vi "N-Parametric Double FFT Mesurament RT.vi"(8 "Triangular Multiply Factor":dbl[](array[numeric])=[1.0, 0.8, 0.95, 0.85, 0.9], 9 "Enable triangular scaling":bool=TRUE, 10 "Triangolo dritto?":bool, 11 "#Signals":u32(slide)=5 scale=1.0..5.0) -> ()   [LabVIEW 2014]
uses:
  <vilib>/Platform/TimedLoop/XDataNode/timing_clust.ctl
  <vilib>/Platform/TimedLoop/XDataNode/nitl_modes.ctl
  <vilib>/Platform/TimedLoop/XDataNode/wakeup.ctl
  <vilib>/FPGAPlugInAG/sbRIO-9636/niLvFpga_Open_sbRIO-9636.vi
  <vilib>/rvi/interface/common/dynamic/niFpgaDynamicAddResources.vi
  <vilib>/FPGAPlugInAG/Dynamic/niLvFpga_Reset_Dynamic.vi
  <vilib>/Utility/error.llb/Error Cluster From Error Code.vi
  <vilib>/rvi/errors/niLvFpgaAdjustHostInterfaceError.vi
  <vilib>/rvi/interface/common/niFpgaWaitOnOcc.vi
  <vilib>/FPGAPlugInAG/Dynamic/niLvFpga_Run_Dynamic.vi
  <vilib>/FPGAPlugInAG/Dynamic/niLvFpga_Abort_Dynamic.vi
  <vilib>/FPGAPlugInAG/Dynamic/niLvFpga_Close_Dynamic.vi
  <vilib>/rvi/interface/nirviOpenFPGA/nirviOpenFPGA.xnode
  FPGA Bitfiles/LaserDistanceSen_FPGATarget_N-ParametricDoub_YVLbjAYtdP4.lvbitx
  FPGA Target/Test VIs/N-Parametric Double FFT Mesurament Test.vi
  FPGA Bitfiles/LaserDistanceSen_FPGATarget_N-ParametricDoub_qx5IM88U9d4.lvbitx
  FPGA Target/Test VIs/N-Parametric Double FFT Mesurament Test SLOW.vi
  <vilib>/rvi/interface/nirviMethod/nirviMethod.xnode
  <vilib>/rvi/interface/nirviReadWriteControl/nirviReadWriteControl.xnode
  <vilib>/Platform/TimedLoop/XDataNode/XDataNode.xnode
  <vilib>/rvi/interface/nirviCloseFPGA/nirviCloseFPGA.xnode
  <vilib>/FPGAPlugInAG/Dynamic/niLvFpga_ConfigureFifo_Dynamic.vi
  <vilib>/rvi/errors/niLvFpgaMergeErrorWithErrorCode.vi
  <vilib>/FPGAPlugInAG/Dynamic/niLvFpga_StartFifo_Dynamic.vi
  <vilib>/rvi/interface/Simulation/niFpgaSimulationCallBeginRW.vi
  <vilib>/FPGAPlugInAG/Dynamic/niLvFpga_ReadFifo_Dynamic.vi
  <vilib>/Platform/TimedLoop/XDataNode/XDNodeRunTimeDep.lvlib
  NiFpgaLv.dll
panel:
  in  "Sample /Modulation Frequency":enum32{"40MHz/32KHz", "30MHz/24Khz"}(radio)
  out "current sig factor":u32
  out "mean factor 1":dbl[](array[numeric])=[1.0, 0.7647004729921506, 0.9587386483466616, 0.823312577391412, 0.8946731320619146]
  out "mean factor 2":dbl[](array[numeric])=[0.9613248197180021, 0.8004726992011919, 0.9202842728499455, 0.8411537208279052, 0.8795877616861416]
  in  "#measure for factor":u32=10
  in  "indice della triangolare a fattore 1":i32
  out "Freq correction factor 1":dbl[](array[numeric])
  out "Freq correction factor 2":dbl[](array[numeric])
  out "Frequencies 2":dbl[](array[numeric])
  out "Frequencies 1":dbl[](array[numeric])
  in  "tieni premuto per":i32=1
  out "Second Std Deviations %":dbl[](array[numeric])
  out "First Std Deviations %":dbl[](array[numeric])
  out "Second Mean Freq Curves":dbl[][](graph)
  out "First Mean Freq Curves":dbl[][](graph)
  in  "# Measurements for Linearization":i32=10
  out "Current Signal":i32
  in  "Linearization?":bool
  out "Second Edge N-FFT":dbl[](graph)
  out "First Edge N-FFT":dbl[](graph)
  in  "stop":bool
  in  "Initial Latency points":u32(slide) scale=0.0..1249.0
  out "Elements Remaining FFT":u32
  out "Elements Remaining Signal":u32
  out "N-Signals":dbl[](graph)
  in  "Snapshot":bool
  in  "Windowing":T1(ring)
  in  "first bin":i32=5
  in  "last bin":i32=255
  in  "lower limit 2":u32(slide)=738 scale=625.0..738.0
  in  "lower limit 1":u32(slide)=113 scale=0.0..113.0
  # "OFFLINE parameters"
  # "WARNING:\nOnce pressed wait untill the end of operation"
  # "Max Detection FFT bin range"
  # "ONLINE parameters"
  # "Calcolo del fattore correttivo di frequenza"
  # "1"
  # "1"
  # "0,82"
  # "0,76"
  # "0,95"
  # "0,96"
  # "0,87"
  # "0,82"
  # "0,91"
  # "0,90"
  # "1st triangular"
  # "2nd triangular"
  # "3rd triangular"
  # "4th triangular"
  # "5th triangular"
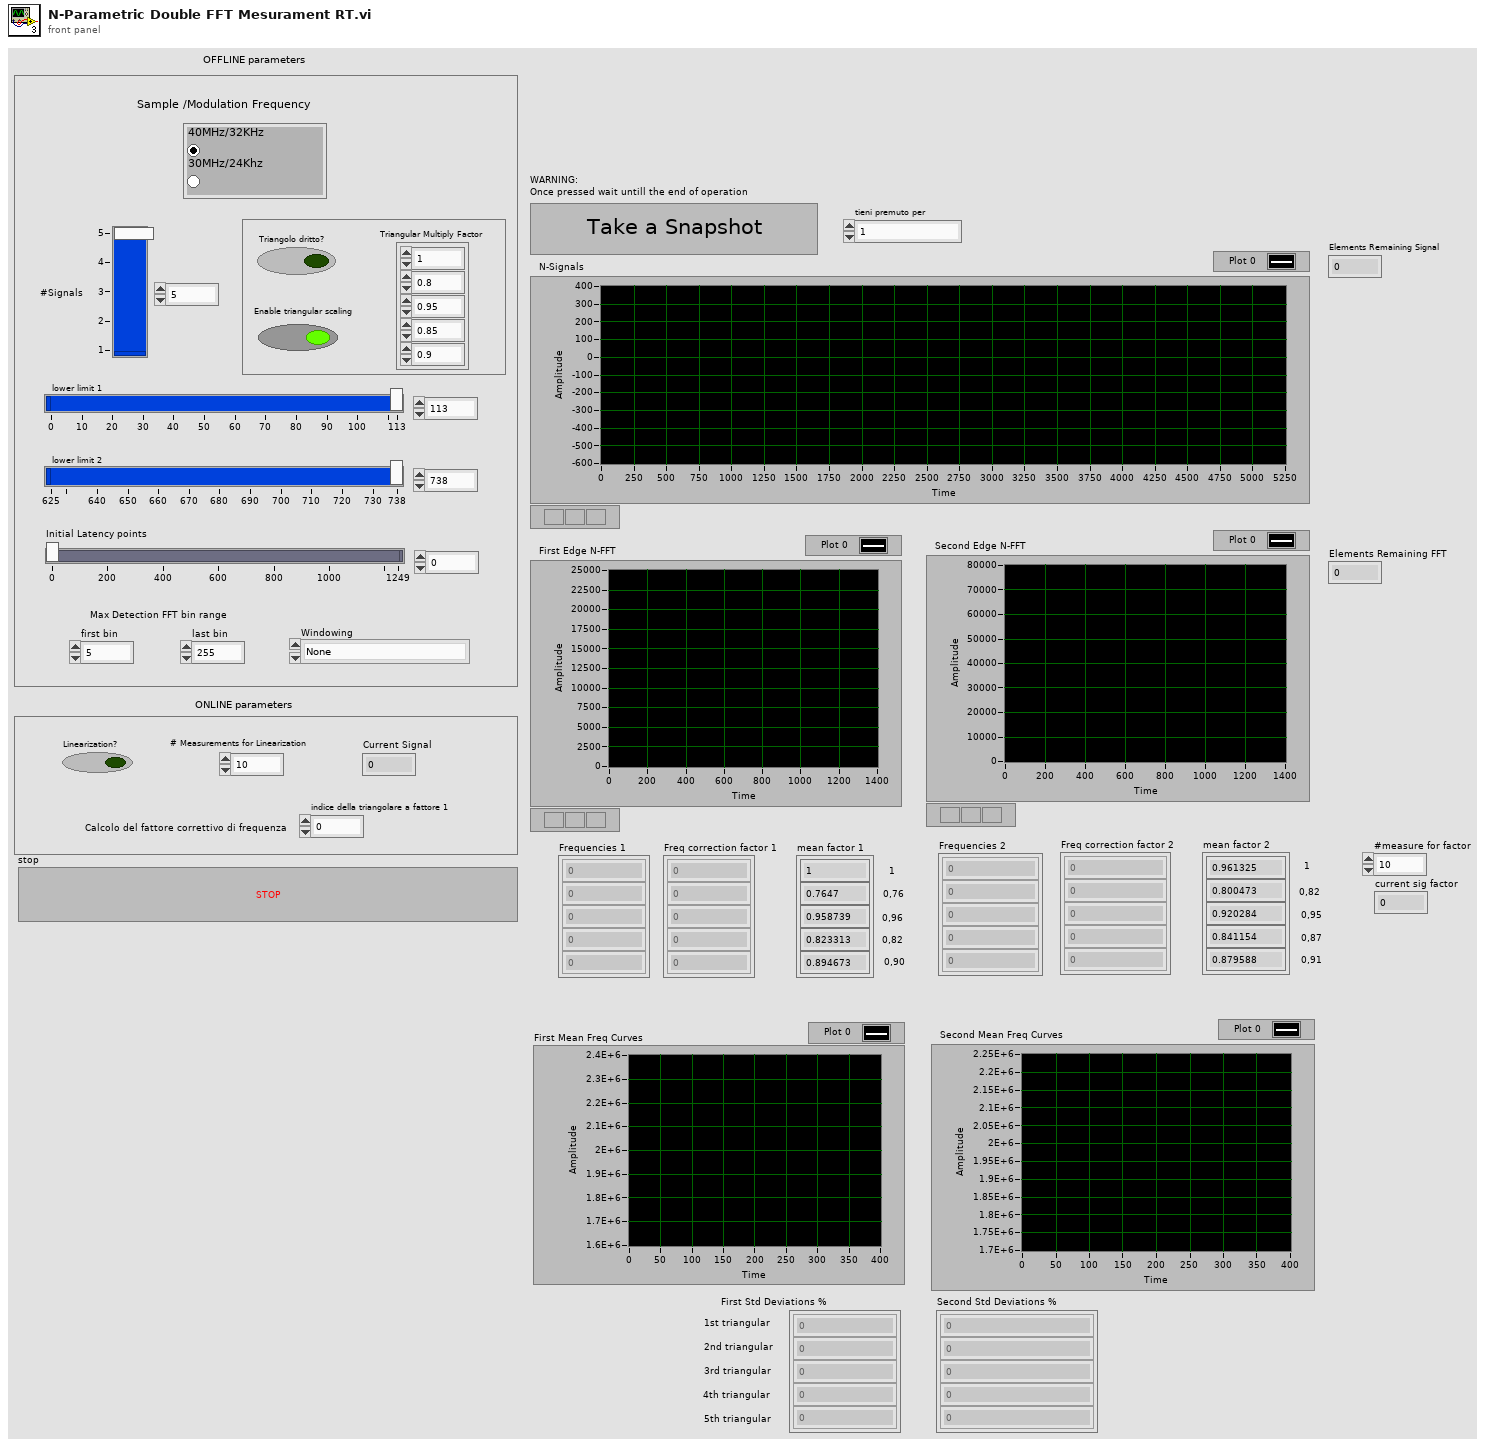
[diagram p1: front panel]
types:
  T1 = enum16{"None", "Hanning", "Hamming", "Blackman", "Blackman-Harris"}
  T2 = typedef "XDNodeRunTimeDep.lvlib/timing_clust.ctl" = cluster{"Expected End [f-1]":u64, "Actual End [f-1]":u64, "Finished Late? [f-1]":bool, "Expected End [i-1]":u64, "Actual End [i-1]":u64, "Finished Late? [i-1]":bool, "Expected Start [i]":u64, "Actual Start [i]":u64, "Expected Start [f]":u64, "Actual Start [f]":u64, "Source Name":string, "Structure Name":string, "Period":i64, "Deadline":i64, "Offset":i64, "Start":i64, "Priority":i32, "Timeout":i32, "Mode":T3, "Wakeup Reason":T4, "Error":errorcluster, "Source Type":string, "Secondary Source Type":string, "Global End Time":u64, "Global Start Time":u64, "Frame Duration":u64, "Iteration Duration":u64, "Assigned CPU":i32, "I/O Scan Engine Mode":u32}
  T3 = typedef "XDNodeRunTimeDep.lvlib/nitl_modes.ctl" = enum32{"No Change", "Process missed periods, maintain original phase", "Discard missed periods, maintain original phase", "Process missed periods, ignore original phase", "Discard missed periods, ignore original phase"}
  T4 = typedef "XDNodeRunTimeDep.lvlib/wakeup.ctl" = enum32{"Normal", "Aborted", "Asynchronous wakeup", "Timing source error", "Timed loop error", "Timeout"}
  T5 = typedef "NI_Matrix.lvlib/RealMatrix.ctl" = dbl[][]
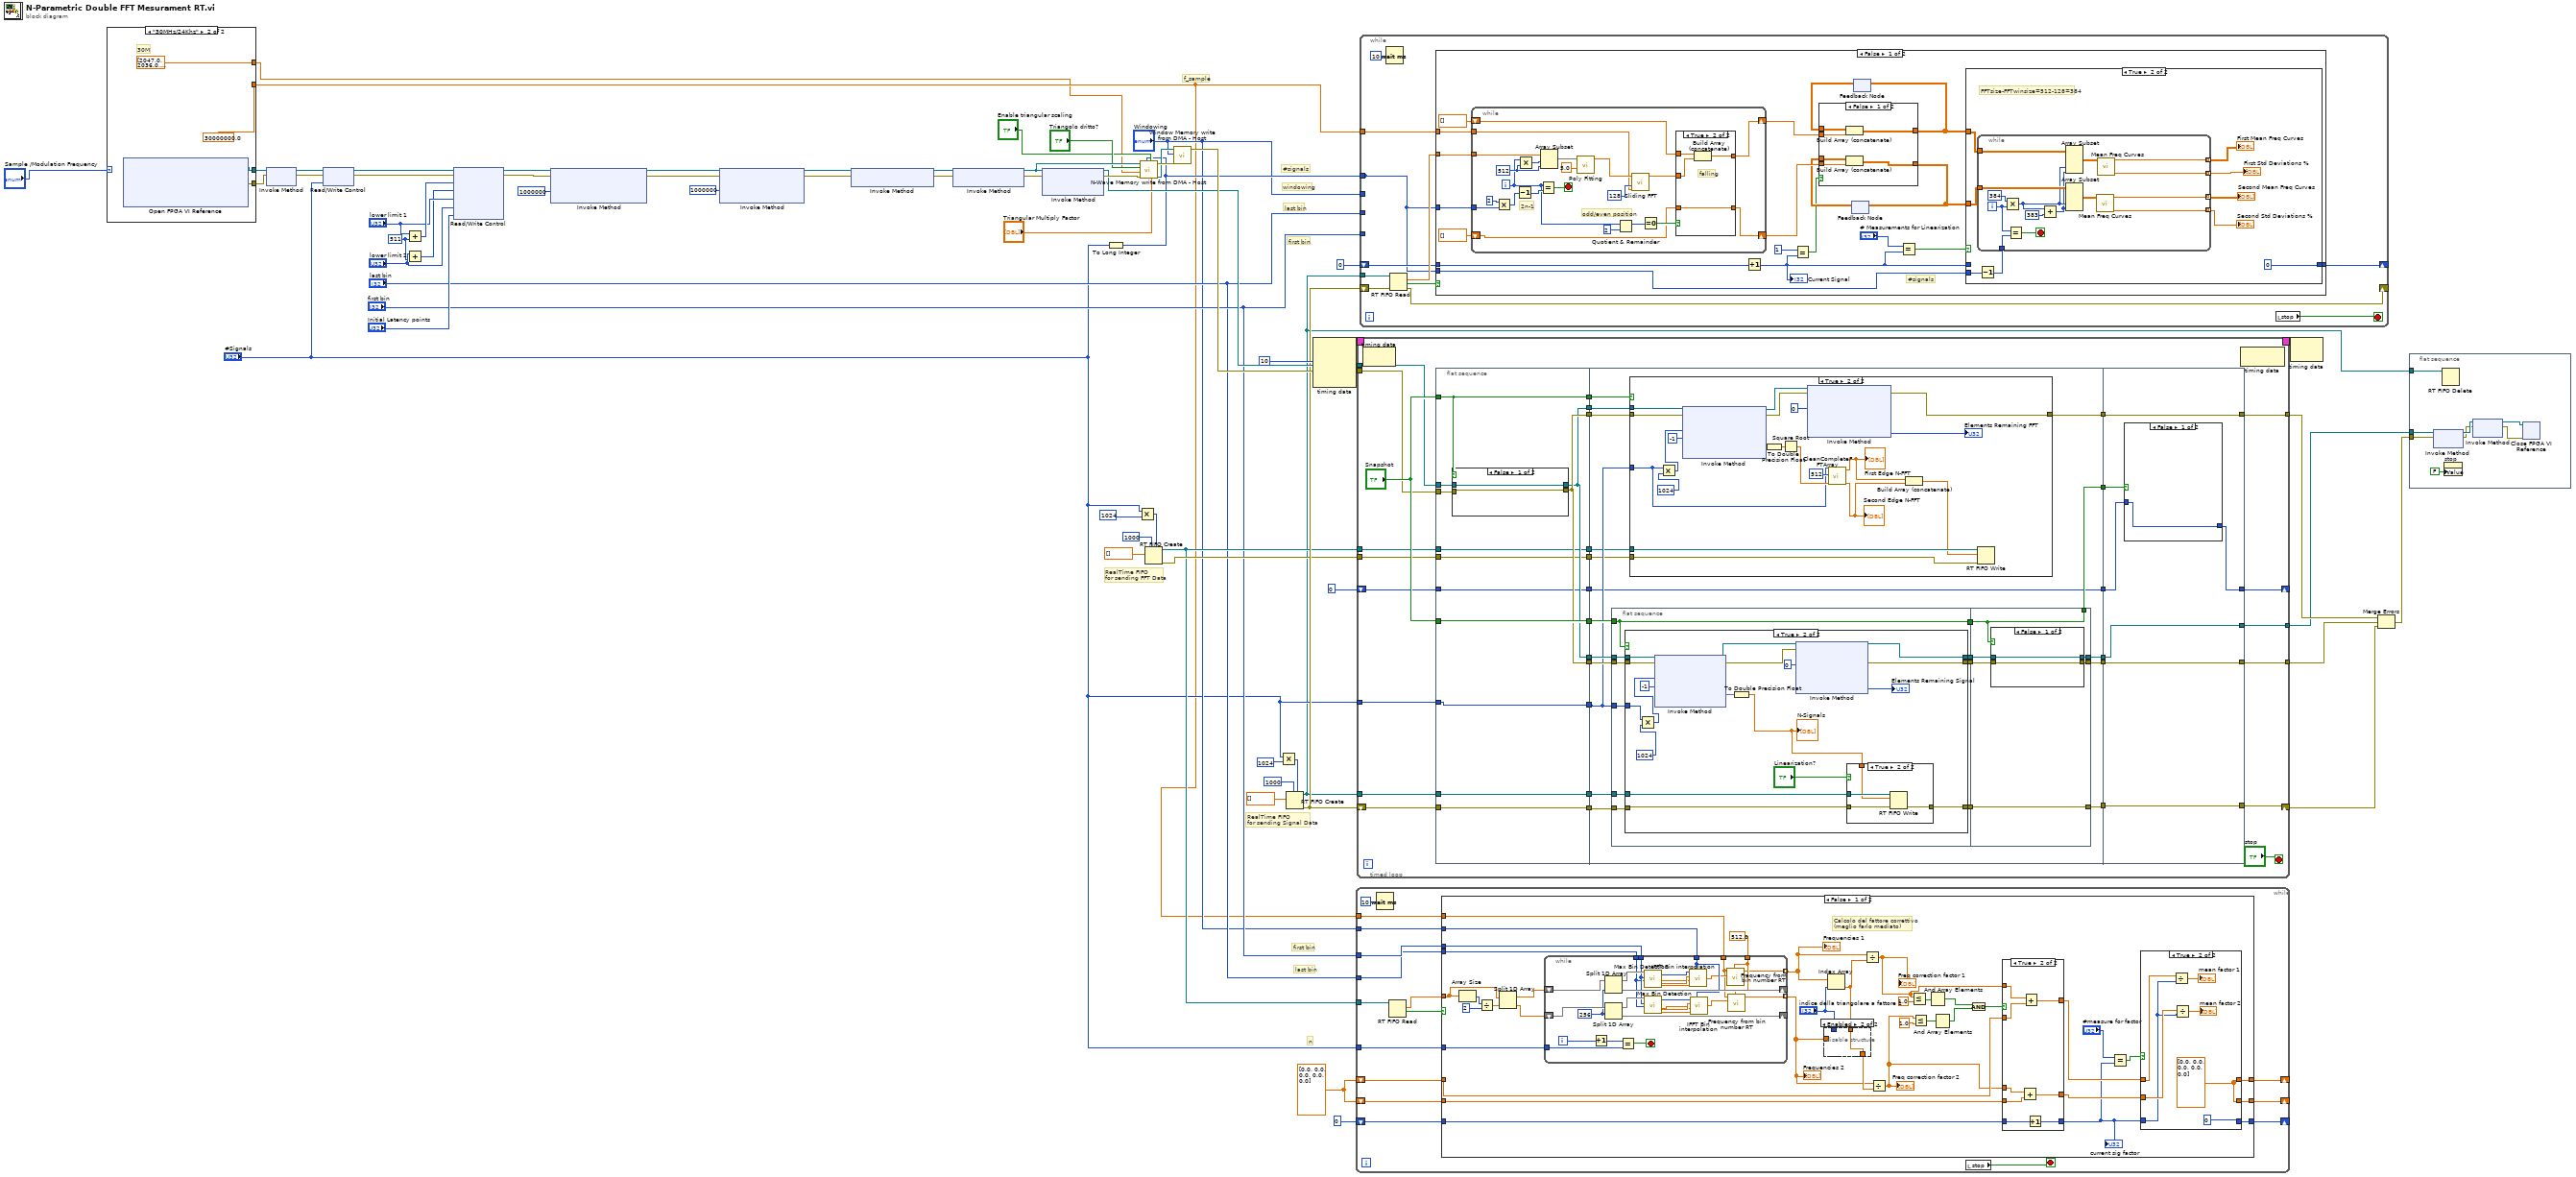
[diagram p0: block diagram]
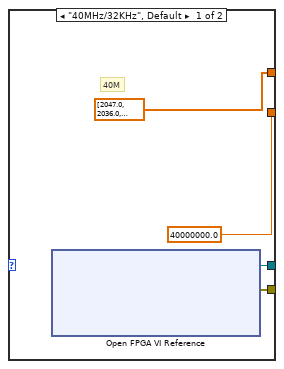
[diagram p2: hidden frame]
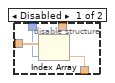
[diagram p3: hidden frame]
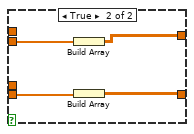
[diagram p8: hidden frame]
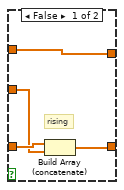
[diagram p9: hidden frame]
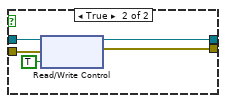
[diagram p11: hidden frame]
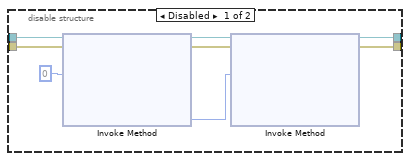
[diagram p13: hidden frame]
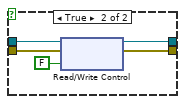
[diagram p15: hidden frame]
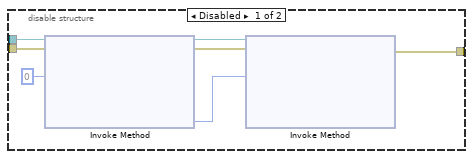
[diagram p17: hidden frame]
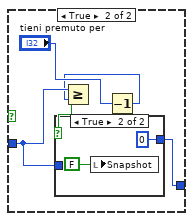
[diagram p18: hidden frame]
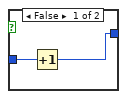
[diagram p19: hidden frame]
diagram:
  w4 = dbl[] [0.0, 0.0, 0.0, 0.0, 0.0] ("second subarray")
  w60 = u32 511 ("y")
  # "n"
  # "last bin"
  # "first bin"
  # "RealTime FIFO \nfor sending FFT Data"
  # "f_sample"
  # "#signals"
  # "RealTime FIFO \nfor sending Signal Data"
  # "windowing"
  # "last bin"
  # "first bin"
  n1 = case shown="\"30MHz/24Khz\"" "Sample /Modulation Frequency" {
    tunnel: [w68 w71] -> w34
    tunnel: [w67 w72] -> w33
    tunnel: [40000000.0 ("Sample Rate (S/s)") 30000000.0 ("Sample Rate (S/s)")] -> w2
    tunnel: [dbl[] [2047.0, 2036.0, 2024.0, 2013.0, 2002.0, 1990.0, 1979.0, 1968.0, 1956.0, 1945.0, 1934.0, 1923.0, 1912.0, 1900.0, 1889.0, 1878.0, 1867.0, 1856.0, 1845.0, 1833.0, 1822.0, 1811.0, 1800.0, 1789.0, 1778.0, 1767.0, 1756.0, 1745.0, 1734.0, 1723.0, 1712.0, 1702.0, 1691.0, 1680.0, 1669.0, 1658.0, 1647.0, 1636.0, 1626.0, 1615.0, 1604.0, 1593.0, 1583.0, 1572.0, 1561.0, 1550.0, 1540.0, 1529.0, 1518.0, 1508.0, 1497.0, 1487.0, 1476.0, 1465.0, 1455.0, 1444.0, 1434.0, 1423.0, 1413.0, 1402.0, 1392.0, 1381.0, 1371.0, 1360.0, 1350.0, 1340.0, 1329.0, 1319.0, 1309.0, 1298.0, 1288.0, 1278.0, 1267.0, 1257.0, 1247.0, 1237.0, 1226.0, 1216.0, 1206.0, 1196.0, 1186.0, 1176.0, 1165.0, 1155.0, 1145.0, 1135.0, 1125.0, 1115.0, 1105.0, 1095.0, 1085.0, 1075.0, 1065.0, 1055.0, 1045.0, 1035.0, 1025.0, 1015.0, 1006.0, 996.0, 986.0, 976.0, 966.0, 956.0, 947.0, 937.0, 927.0, 917.0, 908.0, 898.0, 888.0, 879.0, 869.0, 859.0, 850.0, 837.0, 826.0, 816.0, 804.0, 796.0, 788.0, 778.0, 769.0, 758.0, 750.0, 743.0, 733.0, 724.0, 717.0, 709.0, 701.0, 693.0, 686.0, 677.0, 669.0, 661.0, 653.0, 645.0, 638.0, 630.0, 622.0, 615.0, 607.0, 599.0, 592.0, 583.0, 576.0, 569.0, 561.0, 554.0, 547.0, 539.0, 532.0, 525.0, 518.0, 509.0, 501.0, 492.0, 486.0, 478.0, 471.0, 463.0, 456.0, 450.0, 442.0, 435.0, 429.0, 421.0, 415.0, 408.0, 401.0, 394.0, 388.0, 381.0, 375.0, 368.0, 361.0, 355.0, 349.0, 342.0, 336.0, 330.0, 323.0, 317.0, 311.0, 304.0, 298.0, 292.0, 286.0, 279.0, 273.0, 267.0, 261.0, 255.0, 249.0, 242.0, 236.0, 230.0, 224.0, 218.0, 212.0, 206.0, 200.0, 194.0, 187.0, 181.0, 175.0, 169.0, 163.0, 157.0, 150.0, 144.0, 138.0, 132.0, 125.0, 119.0, 113.0, 107.0, 101.0, 95.0, 88.0, 82.0, 77.0, 71.0, 65.0, 59.0, 53.0, 47.0, 41.0, 35.0, 29.0, 23.0, 18.0, 11.0, 6.0, 0.0, -6.0, -12.0, -18.0, -23.0, -29.0, -35.0, -41.0, -47.0, -52.0, -58.0, -64.0, -69.0, -75.0, -81.0, -87.0, -92.0, -98.0, -104.0, -109.0, -115.0, -121.0, -126.0, -132.0, -138.0, -144.0, -149.0, -155.0, -161.0, -166.0, -172.0, -177.0, -183.0, -189.0, -194.0, -200.0, -205.0, -211.0, -216.0, -222.0, -227.0, -233.0, -238.0, -244.0, -249.0, -255.0, -260.0, -266.0, -271.0, -277.0, -283.0, -288.0, -294.0, -299.0, -304.0, -310.0, -315.0, -321.0, -326.0, -331.0, -337.0, -342.0, -348.0, -353.0, -358.0, -364.0, -369.0, -375.0, -380.0, -385.0, -391.0, -396.0, -402.0, -407.0, -413.0, -418.0, -423.0, -429.0, -434.0, -439.0, -445.0, -450.0, -456.0, -461.0, -466.0, -472.0, -477.0, -483.0, -488.0, -493.0, -499.0, -504.0, -510.0, -515.0, -520.0, -526.0, -531.0, -537.0, -542.0, -548.0, -553.0, -558.0, -564.0, -569.0, -574.0, -580.0, -585.0, -590.0, -596.0, -601.0, -606.0, -612.0, -617.0, -622.0, -628.0, -633.0, -638.0, -644.0, -649.0, -654.0, -660.0, -665.0, -670.0, -676.0, -681.0, -686.0, -692.0, -697.0, -702.0, -708.0, -713.0, -718.0, -723.0, -729.0, -734.0, -739.0, -744.0, -750.0, -755.0, -760.0, -765.0, -771.0, -776.0, -781.0, -786.0, -792.0, -797.0, -802.0, -807.0, -812.0, -818.0, -823.0, -828.0, -833.0, -839.0, -844.0, -849.0, -854.0, -859.0, -865.0, -870.0, -875.0, -880.0, -885.0, -891.0, -896.0, -901.0, -906.0, -911.0, -916.0, -922.0, -927.0, -932.0, -937.0, -943.0, -948.0, -953.0, -958.0, -963.0, -969.0, -974.0, -979.0, -984.0, -989.0, -995.0, -1000.0, -1005.0, -1010.0, -1015.0, -1021.0, -1026.0, -1031.0, -1036.0, -1041.0, -1047.0, -1052.0, -1057.0, -1062.0, -1067.0, -1073.0, -1078.0, -1083.0, -1088.0, -1093.0, -1099.0, -1104.0, -1109.0, -1114.0, -1119.0, -1124.0, -1130.0, -1135.0, -1140.0, -1145.0, -1150.0, -1156.0, -1161.0, -1166.0, -1171.0, -1176.0, -1182.0, -1187.0, -1192.0, -1197.0, -1202.0, -1207.0, -1213.0, -1218.0, -1223.0, -1228.0, -1233.0, -1238.0, -1244.0, -1249.0, -1254.0, -1259.0, -1264.0, -1269.0, -1275.0, -1280.0, -1285.0, -1290.0, -1295.0, -1300.0, -1305.0, -1311.0, -1316.0, -1321.0, -1326.0, -1331.0, -1336.0, -1342.0, -1347.0, -1352.0, -1357.0, -1362.0, -1367.0, -1372.0, -1378.0, -1383.0, -1388.0, -1393.0, -1398.0, -1403.0, -1408.0, -1414.0, -1419.0, -1424.0, -1429.0, -1434.0, -1439.0, -1444.0, -1450.0, -1455.0, -1460.0, -1465.0, -1470.0, -1475.0, -1480.0, -1486.0, -1491.0, -1496.0, -1501.0, -1506.0, -1511.0, -1516.0, -1522.0, -1527.0, -1532.0, -1537.0, -1542.0, -1547.0, -1552.0, -1558.0, -1563.0, -1568.0, -1573.0, -1578.0, -1583.0, -1588.0, -1593.0, -1599.0, -1604.0, -1609.0, -1614.0, -1619.0, -1624.0, -1629.0, -1634.0, -1640.0, -1645.0, -1650.0, -1655.0, -1660.0, -1665.0, -1670.0, -1675.0, -1681.0, -1686.0, -1691.0, -1696.0, -1701.0, -1706.0, -1711.0, -1716.0, -1722.0, -1727.0, -1732.0, -1737.0, -1742.0, -1747.0, -1752.0, -1757.0, -1762.0, -1768.0, -1773.0, -1778.0, -1783.0, -1788.0, -1793.0, -1798.0, -1803.0, -1808.0, -1814.0, -1819.0, -1824.0, -1829.0, -1834.0, -1839.0, -1844.0, -1849.0, -1854.0, -1859.0, -1865.0, -1870.0, -1875.0, -1880.0, -1885.0, -1890.0, -1895.0, -1900.0, -1905.0, -1911.0, -1916.0, -1921.0, -1926.0, -1931.0, -1936.0, -1941.0, -1946.0, -1951.0, -1956.0, -1961.0, -1967.0, -1972.0, -1977.0, -1982.0, -1987.0, -1992.0, -1997.0, -2002.0, -2007.0, -2012.0, -2017.0, -2023.0, -2028.0, -2033.0, -2038.0, -2043.0, -2048.0, -2047.0, -2034.0, -2021.0, -2009.0, -1996.0, -1983.0, -1970.0, -1957.0, -1945.0, -1932.0, -1919.0, -1907.0, -1894.0, -1881.0, -1869.0, -1856.0, -1844.0, -1831.0, -1819.0, -1806.0, -1794.0, -1781.0, -1769.0, -1757.0, -1744.0, -1732.0, -1719.0, -1707.0, -1695.0, -1682.0, -1670.0, -1658.0, -1646.0, -1634.0, -1621.0, -1609.0, -1597.0, -1585.0, -1573.0, -1561.0, -1549.0, -1537.0, -1525.0, -1513.0, -1501.0, -1489.0, -1477.0, -1465.0, -1453.0, -1441.0, -1429.0, -1417.0, -1405.0, -1394.0, -1382.0, -1370.0, -1358.0, -1347.0, -1335.0, -1323.0, -1312.0, -1300.0, -1288.0, -1277.0, -1265.0, -1254.0, -1242.0, -1231.0, -1219.0, -1208.0, -1196.0, -1185.0, -1173.0, -1162.0, -1150.0, -1139.0, -1128.0, -1116.0, -1105.0, -1094.0, -1083.0, -1071.0, -1060.0, -1049.0, -1038.0, -1027.0, -1015.0, -1004.0, -993.0, -982.0, -971.0, -960.0, -949.0, -938.0, -927.0, -916.0, -905.0, -894.0, -883.0, -873.0, -862.0, -851.0, -840.0, -829.0, -819.0, -808.0, -797.0, -786.0, -776.0, -765.0, -754.0, -744.0, -733.0, -722.0, -712.0, -697.0, -685.0, -674.0, -661.0, -652.0, -643.0, -632.0, -622.0, -610.0, -602.0, -594.0, -583.0, -574.0, -566.0, -558.0, -550.0, -542.0, -534.0, -525.0, -516.0, -507.0, -499.0, -491.0, -483.0, -475.0, -467.0, -459.0, -451.0, -443.0, -435.0, -426.0, -419.0, -411.0, -404.0, -396.0, -388.0, -381.0, -373.0, -366.0, -359.0, -349.0, -341.0, -331.0, -325.0, -317.0, -309.0, -301.0, -295.0, -288.0, -280.0, -273.0, -266.0, -259.0, -252.0, -246.0, -239.0, -231.0, -225.0, -219.0, -212.0, -205.0, -199.0, -192.0, -186.0, -180.0, -173.0, -167.0, -161.0, -155.0, -148.0, -142.0, -136.0, -130.0, -124.0, -118.0, -112.0, -106.0, -100.0, -94.0, -88.0, -82.0, -76.0, -70.0, -64.0, -58.0, -52.0, -46.0, -40.0, -34.0, -28.0, -21.0, -15.0, -9.0, -3.0, 2.0, 9.0, 15.0, 21.0, 27.0, 33.0, 39.0, 45.0, 51.0, 57.0, 63.0, 69.0, 75.0, 81.0, 86.0, 92.0, 98.0, 103.0, 110.0, 116.0, 121.0, 127.0, 133.0, 138.0, 144.0, 149.0, 155.0, 161.0, 166.0, 172.0, 177.0, 183.0, 189.0, 194.0, 200.0, 205.0, 211.0, 216.0, 221.0, 227.0, 232.0, 238.0, 243.0, 249.0, 254.0, 259.0, 265.0, 270.0, 276.0, 281.0, 286.0, 292.0, 297.0, 303.0, 308.0, 314.0, 319.0, 324.0, 329.0, 335.0, 340.0, 345.0, 351.0, 356.0, 361.0, 366.0, 371.0, 377.0, 382.0, 387.0, 392.0, 397.0, 403.0, 408.0, 413.0, 418.0, 423.0, 429.0, 434.0, 439.0, 444.0, 449.0, 454.0, 459.0, 464.0, 469.0, 474.0, 479.0, 484.0, 489.0, 494.0, 499.0, 504.0, 509.0, 514.0, 520.0, 525.0, 530.0, 535.0, 540.0, 545.0, 550.0, 555.0, 560.0, 565.0, 570.0, 575.0, 580.0, 585.0, 590.0, 595.0, 600.0, 605.0, 610.0, 615.0, 620.0, 625.0, 630.0, 636.0, 641.0, 646.0, 651.0, 656.0, 661.0, 666.0, 671.0, 676.0, 681.0, 686.0, 691.0, 696.0, 701.0, 706.0, 711.0, 716.0, 721.0, 726.0, 731.0, 736.0, 741.0, 746.0, 751.0, 756.0, 761.0, 765.0, 770.0, 775.0, 780.0, 785.0, 790.0, 795.0, 800.0, 805.0, 810.0, 815.0, 820.0, 825.0, 829.0, 834.0, 839.0, 844.0, 849.0, 854.0, 859.0, 864.0, 868.0, 873.0, 878.0, 883.0, 888.0, 893.0, 897.0, 902.0, 907.0, 912.0, 917.0, 921.0, 926.0, 931.0, 936.0, 941.0, 945.0, 950.0, 955.0, 960.0, 965.0, 969.0, 974.0, 979.0, 984.0, 988.0, 993.0, 998.0, 1003.0, 1007.0, 1012.0, 1017.0, 1022.0, 1027.0, 1031.0, 1036.0, 1041.0, 1046.0, 1051.0, 1055.0, 1060.0, 1065.0, 1070.0, 1075.0, 1079.0, 1084.0, 1089.0, 1094.0, 1098.0, 1103.0, 1108.0, 1113.0, 1118.0, 1122.0, 1127.0, 1132.0, 1137.0, 1141.0, 1146.0, 1151.0, 1156.0, 1161.0, 1165.0, 1170.0, 1175.0, 1180.0, 1184.0, 1189.0, 1194.0, 1199.0, 1204.0, 1208.0, 1213.0, 1218.0, 1223.0, 1227.0, 1232.0, 1237.0, 1242.0, 1246.0, 1251.0, 1256.0, 1261.0, 1265.0, 1270.0, 1275.0, 1280.0, 1284.0, 1289.0, 1294.0, 1299.0, 1303.0, 1308.0, 1313.0, 1318.0, 1322.0, 1327.0, 1332.0, 1336.0, 1341.0, 1346.0, 1351.0, 1355.0, 1360.0, 1365.0, 1370.0, 1374.0, 1379.0, 1384.0, 1388.0, 1393.0, 1398.0, 1403.0, 1407.0, 1412.0, 1417.0, 1421.0, 1426.0, 1431.0, 1436.0, 1440.0, 1445.0, 1450.0, 1454.0, 1459.0, 1464.0, 1469.0, 1473.0, 1478.0, 1483.0, 1487.0, 1492.0, 1497.0, 1502.0, 1506.0, 1511.0, 1516.0, 1520.0, 1525.0, 1530.0, 1535.0, 1539.0, 1544.0, 1549.0, 1553.0, 1558.0, 1563.0, 1567.0, 1572.0, 1577.0, 1582.0, 1586.0, 1591.0, 1596.0, 1600.0, 1605.0, 1610.0, 1614.0, 1619.0, 1624.0, 1628.0, 1633.0, 1638.0, 1643.0, 1647.0, 1652.0, 1657.0, 1661.0, 1666.0, 1671.0, 1675.0, 1680.0, 1685.0, 1689.0, 1694.0, 1699.0, 1703.0, 1708.0, 1713.0, 1717.0, 1722.0, 1727.0, 1731.0, 1736.0, 1741.0, 1746.0, 1750.0, 1755.0, 1760.0, 1764.0, 1769.0, 1774.0, 1778.0, 1783.0, 1788.0, 1792.0, 1797.0, 1802.0, 1806.0, 1811.0, 1816.0, 1820.0, 1825.0, 1830.0, 1834.0, 1839.0, 1844.0, 1848.0, 1853.0, 1858.0, 1862.0, 1867.0, 1871.0, 1876.0, 1881.0, 1885.0, 1890.0, 1895.0, 1899.0, 1904.0, 1909.0, 1913.0, 1918.0, 1923.0, 1927.0, 1932.0, 1937.0, 1941.0, 1946.0, 1951.0, 1955.0, 1960.0, 1965.0, 1969.0, 1974.0, 1978.0, 1983.0, 1988.0, 1992.0, 1997.0, 2002.0, 2006.0, 2011.0, 2016.0, 2020.0, 2025.0, 2029.0, 2034.0, 2039.0, 2043.0, 2048.0] ("Complete SkewTri") dbl[] [2047.0, 2036.0, 2026.0, 2015.0, 2004.0, 1993.0, 1983.0, 1972.0, 1961.0, 1951.0, 1940.0, 1930.0, 1919.0, 1908.0, 1898.0, 1887.0, 1877.0, 1866.0, 1856.0, 1845.0, 1835.0, 1824.0, 1814.0, 1803.0, 1793.0, 1783.0, 1772.0, 1762.0, 1751.0, 1741.0, 1731.0, 1720.0, 1710.0, 1700.0, 1690.0, 1679.0, 1669.0, 1659.0, 1648.0, 1638.0, 1628.0, 1618.0, 1608.0, 1597.0, 1587.0, 1577.0, 1567.0, 1557.0, 1547.0, 1537.0, 1527.0, 1517.0, 1507.0, 1496.0, 1486.0, 1476.0, 1466.0, 1456.0, 1446.0, 1437.0, 1427.0, 1417.0, 1407.0, 1397.0, 1387.0, 1377.0, 1367.0, 1357.0, 1348.0, 1338.0, 1328.0, 1318.0, 1308.0, 1299.0, 1289.0, 1279.0, 1269.0, 1260.0, 1250.0, 1240.0, 1230.0, 1221.0, 1211.0, 1202.0, 1192.0, 1182.0, 1173.0, 1163.0, 1154.0, 1144.0, 1134.0, 1125.0, 1115.0, 1106.0, 1096.0, 1087.0, 1077.0, 1068.0, 1059.0, 1049.0, 1040.0, 1030.0, 1021.0, 1012.0, 1002.0, 993.0, 984.0, 974.0, 965.0, 956.0, 946.0, 937.0, 928.0, 919.0, 909.0, 900.0, 891.0, 882.0, 873.0, 862.0, 853.0, 845.0, 836.0, 827.0, 816.0, 806.0, 797.0, 786.0, 778.0, 769.0, 759.0, 750.0, 742.0, 734.0, 725.0, 717.0, 708.0, 699.0, 691.0, 683.0, 675.0, 668.0, 660.0, 652.0, 645.0, 637.0, 629.0, 622.0, 614.0, 607.0, 599.0, 592.0, 584.0, 577.0, 570.0, 562.0, 555.0, 548.0, 541.0, 534.0, 526.0, 519.0, 512.0, 505.0, 498.0, 491.0, 484.0, 477.0, 470.0, 463.0, 457.0, 449.0, 443.0, 436.0, 429.0, 422.0, 415.0, 409.0, 402.0, 395.0, 388.0, 381.0, 374.0, 367.0, 361.0, 354.0, 347.0, 340.0, 334.0, 327.0, 321.0, 314.0, 308.0, 301.0, 295.0, 288.0, 282.0, 276.0, 269.0, 263.0, 257.0, 251.0, 244.0, 238.0, 232.0, 226.0, 220.0, 213.0, 207.0, 201.0, 195.0, 189.0, 183.0, 177.0, 171.0, 164.0, 158.0, 152.0, 146.0, 140.0, 134.0, 128.0, 122.0, 116.0, 110.0, 104.0, 98.0, 92.0, 86.0, 80.0, 74.0, 68.0, 62.0, 56.0, 50.0, 44.0, 38.0, 32.0, 26.0, 20.0, 15.0, 9.0, 3.0, -3.0, -9.0, -15.0, -21.0, -27.0, -32.0, -38.0, -44.0, -50.0, -56.0, -61.0, -67.0, -73.0, -79.0, -85.0, -90.0, -96.0, -102.0, -108.0, -114.0, -119.0, -125.0, -131.0, -137.0, -142.0, -148.0, -154.0, -159.0, -165.0, -171.0, -176.0, -182.0, -188.0, -193.0, -199.0, -205.0, -210.0, -216.0, -222.0, -227.0, -233.0, -239.0, -244.0, -250.0, -256.0, -261.0, -267.0, -272.0, -278.0, -284.0, -289.0, -295.0, -300.0, -306.0, -311.0, -317.0, -323.0, -328.0, -334.0, -340.0, -345.0, -351.0, -356.0, -362.0, -368.0, -373.0, -379.0, -384.0, -390.0, -395.0, -401.0, -407.0, -412.0, -418.0, -423.0, -429.0, -434.0, -440.0, -445.0, -451.0, -456.0, -462.0, -467.0, -473.0, -478.0, -484.0, -489.0, -495.0, -501.0, -506.0, -512.0, -517.0, -523.0, -528.0, -533.0, -539.0, -544.0, -550.0, -555.0, -561.0, -566.0, -572.0, -577.0, -583.0, -588.0, -594.0, -599.0, -604.0, -610.0, -615.0, -621.0, -626.0, -632.0, -637.0, -642.0, -648.0, -653.0, -659.0, -664.0, -669.0, -675.0, -680.0, -686.0, -691.0, -696.0, -702.0, -707.0, -712.0, -718.0, -723.0, -729.0, -734.0, -739.0, -745.0, -750.0, -755.0, -761.0, -766.0, -771.0, -777.0, -782.0, -787.0, -793.0, -798.0, -803.0, -809.0, -814.0, -819.0, -825.0, -830.0, -835.0, -841.0, -846.0, -851.0, -857.0, -862.0, -868.0, -873.0, -878.0, -884.0, -889.0, -894.0, -900.0, -905.0, -910.0, -916.0, -921.0, -926.0, -932.0, -937.0, -942.0, -947.0, -953.0, -958.0, -963.0, -969.0, -974.0, -979.0, -985.0, -990.0, -995.0, -1001.0, -1006.0, -1011.0, -1017.0, -1022.0, -1027.0, -1033.0, -1038.0, -1043.0, -1048.0, -1054.0, -1059.0, -1064.0, -1070.0, -1075.0, -1080.0, -1086.0, -1091.0, -1096.0, -1102.0, -1107.0, -1112.0, -1118.0, -1123.0, -1128.0, -1134.0, -1139.0, -1144.0, -1149.0, -1155.0, -1160.0, -1165.0, -1171.0, -1176.0, -1181.0, -1186.0, -1192.0, -1197.0, -1202.0, -1208.0, -1213.0, -1218.0, -1223.0, -1229.0, -1234.0, -1239.0, -1245.0, -1250.0, -1255.0, -1260.0, -1266.0, -1271.0, -1276.0, -1281.0, -1287.0, -1292.0, -1297.0, -1302.0, -1308.0, -1313.0, -1318.0, -1323.0, -1329.0, -1334.0, -1339.0, -1344.0, -1350.0, -1355.0, -1360.0, -1365.0, -1371.0, -1376.0, -1381.0, -1386.0, -1392.0, -1397.0, -1402.0, -1407.0, -1412.0, -1418.0, -1423.0, -1428.0, -1433.0, -1439.0, -1444.0, -1449.0, -1454.0, -1460.0, -1465.0, -1470.0, -1475.0, -1480.0, -1486.0, -1491.0, -1496.0, -1501.0, -1507.0, -1512.0, -1517.0, -1522.0, -1528.0, -1533.0, -1538.0, -1543.0, -1548.0, -1554.0, -1559.0, -1564.0, -1569.0, -1575.0, -1580.0, -1585.0, -1590.0, -1595.0, -1601.0, -1606.0, -1611.0, -1616.0, -1622.0, -1627.0, -1632.0, -1637.0, -1642.0, -1648.0, -1653.0, -1658.0, -1663.0, -1668.0, -1674.0, -1679.0, -1684.0, -1689.0, -1695.0, -1700.0, -1705.0, -1710.0, -1715.0, -1721.0, -1726.0, -1731.0, -1736.0, -1741.0, -1747.0, -1752.0, -1757.0, -1762.0, -1767.0, -1773.0, -1778.0, -1783.0, -1788.0, -1793.0, -1799.0, -1804.0, -1809.0, -1814.0, -1819.0, -1825.0, -1830.0, -1835.0, -1840.0, -1845.0, -1851.0, -1856.0, -1861.0, -1866.0, -1871.0, -1877.0, -1882.0, -1887.0, -1892.0, -1897.0, -1903.0, -1908.0, -1913.0, -1918.0, -1923.0, -1929.0, -1934.0, -1939.0, -1944.0, -1949.0, -1955.0, -1960.0, -1965.0, -1970.0, -1975.0, -1981.0, -1986.0, -1991.0, -1996.0, -2001.0, -2007.0, -2012.0, -2017.0, -2022.0, -2027.0, -2032.0, -2038.0, -2043.0, -2048.0, -2047.0, -2035.0, -2022.0, -2010.0, -1997.0, -1985.0, -1973.0, -1960.0, -1948.0, -1936.0, -1923.0, -1911.0, -1899.0, -1887.0, -1874.0, -1862.0, -1850.0, -1838.0, -1826.0, -1814.0, -1801.0, -1789.0, -1777.0, -1765.0, -1753.0, -1741.0, -1729.0, -1717.0, -1705.0, -1693.0, -1681.0, -1670.0, -1658.0, -1646.0, -1634.0, -1622.0, -1610.0, -1599.0, -1587.0, -1575.0, -1563.0, -1552.0, -1540.0, -1528.0, -1517.0, -1505.0, -1494.0, -1482.0, -1470.0, -1459.0, -1447.0, -1436.0, -1424.0, -1413.0, -1401.0, -1390.0, -1378.0, -1367.0, -1356.0, -1344.0, -1333.0, -1322.0, -1310.0, -1299.0, -1288.0, -1277.0, -1265.0, -1254.0, -1243.0, -1232.0, -1221.0, -1209.0, -1198.0, -1187.0, -1176.0, -1165.0, -1154.0, -1143.0, -1132.0, -1121.0, -1110.0, -1099.0, -1088.0, -1077.0, -1066.0, -1056.0, -1045.0, -1034.0, -1023.0, -1012.0, -1002.0, -991.0, -980.0, -969.0, -959.0, -948.0, -937.0, -927.0, -916.0, -905.0, -895.0, -884.0, -874.0, -863.0, -853.0, -842.0, -832.0, -821.0, -811.0, -800.0, -790.0, -780.0, -769.0, -759.0, -749.0, -738.0, -729.0, -718.0, -710.0, -701.0, -692.0, -683.0, -675.0, -666.0, -658.0, -650.0, -642.0, -634.0, -626.0, -618.0, -610.0, -602.0, -594.0, -586.0, -578.0, -570.0, -563.0, -555.0, -547.0, -540.0, -532.0, -524.0, -517.0, -510.0, -502.0, -495.0, -487.0, -480.0, -473.0, -466.0, -457.0, -450.0, -442.0, -435.0, -428.0, -420.0, -413.0, -406.0, -399.0, -391.0, -384.0, -377.0, -370.0, -363.0, -356.0, -349.0, -342.0, -336.0, -329.0, -323.0, -316.0, -310.0, -304.0, -297.0, -291.0, -285.0, -278.0, -272.0, -266.0, -260.0, -254.0, -247.0, -241.0, -235.0, -229.0, -223.0, -216.0, -210.0, -204.0, -198.0, -192.0, -186.0, -180.0, -173.0, -167.0, -161.0, -155.0, -149.0, -143.0, -136.0, -130.0, -124.0, -118.0, -112.0, -106.0, -100.0, -94.0, -88.0, -82.0, -76.0, -70.0, -64.0, -58.0, -51.0, -45.0, -39.0, -33.0, -27.0, -21.0, -15.0, -9.0, -3.0, 3.0, 9.0, 15.0, 21.0, 26.0, 32.0, 38.0, 44.0, 49.0, 55.0, 61.0, 66.0, 72.0, 77.0, 83.0, 89.0, 94.0, 100.0, 105.0, 111.0, 116.0, 122.0, 128.0, 133.0, 139.0, 144.0, 150.0, 155.0, 161.0, 166.0, 172.0, 177.0, 183.0, 188.0, 193.0, 199.0, 204.0, 210.0, 215.0, 221.0, 226.0, 232.0, 237.0, 242.0, 248.0, 253.0, 259.0, 264.0, 269.0, 275.0, 280.0, 286.0, 291.0, 297.0, 302.0, 307.0, 313.0, 318.0, 324.0, 329.0, 334.0, 340.0, 345.0, 351.0, 356.0, 361.0, 367.0, 372.0, 378.0, 383.0, 388.0, 394.0, 399.0, 404.0, 410.0, 415.0, 421.0, 426.0, 431.0, 437.0, 442.0, 448.0, 453.0, 458.0, 464.0, 469.0, 474.0, 480.0, 485.0, 490.0, 495.0, 501.0, 506.0, 511.0, 516.0, 522.0, 527.0, 532.0, 537.0, 543.0, 548.0, 553.0, 558.0, 563.0, 569.0, 574.0, 579.0, 584.0, 589.0, 595.0, 600.0, 605.0, 610.0, 615.0, 621.0, 626.0, 631.0, 636.0, 641.0, 646.0, 651.0, 657.0, 662.0, 667.0, 672.0, 677.0, 682.0, 687.0, 693.0, 698.0, 703.0, 708.0, 713.0, 718.0, 723.0, 729.0, 734.0, 739.0, 744.0, 749.0, 754.0, 759.0, 764.0, 769.0, 775.0, 780.0, 785.0, 790.0, 795.0, 800.0, 805.0, 810.0, 815.0, 821.0, 826.0, 831.0, 836.0, 841.0, 846.0, 851.0, 856.0, 861.0, 866.0, 871.0, 877.0, 882.0, 887.0, 892.0, 897.0, 902.0, 907.0, 912.0, 917.0, 922.0, 927.0, 932.0, 937.0, 942.0, 947.0, 952.0, 958.0, 963.0, 968.0, 973.0, 978.0, 983.0, 988.0, 993.0, 998.0, 1003.0, 1008.0, 1013.0, 1018.0, 1023.0, 1028.0, 1033.0, 1038.0, 1043.0, 1048.0, 1053.0, 1058.0, 1063.0, 1068.0, 1073.0, 1078.0, 1083.0, 1088.0, 1093.0, 1098.0, 1103.0, 1108.0, 1113.0, 1118.0, 1123.0, 1128.0, 1133.0, 1138.0, 1143.0, 1148.0, 1153.0, 1158.0, 1163.0, 1168.0, 1173.0, 1178.0, 1183.0, 1188.0, 1193.0, 1198.0, 1203.0, 1208.0, 1213.0, 1218.0, 1223.0, 1228.0, 1233.0, 1238.0, 1243.0, 1248.0, 1253.0, 1258.0, 1263.0, 1268.0, 1273.0, 1277.0, 1282.0, 1287.0, 1292.0, 1297.0, 1302.0, 1307.0, 1312.0, 1317.0, 1322.0, 1327.0, 1332.0, 1337.0, 1342.0, 1347.0, 1352.0, 1357.0, 1362.0, 1367.0, 1371.0, 1376.0, 1381.0, 1386.0, 1391.0, 1396.0, 1401.0, 1406.0, 1411.0, 1416.0, 1421.0, 1426.0, 1431.0, 1435.0, 1440.0, 1445.0, 1450.0, 1455.0, 1460.0, 1465.0, 1470.0, 1475.0, 1480.0, 1485.0, 1489.0, 1494.0, 1499.0, 1504.0, 1509.0, 1514.0, 1519.0, 1524.0, 1529.0, 1534.0, 1538.0, 1543.0, 1548.0, 1553.0, 1558.0, 1563.0, 1568.0, 1573.0, 1578.0, 1582.0, 1587.0, 1592.0, 1597.0, 1602.0, 1607.0, 1612.0, 1617.0, 1622.0, 1626.0, 1631.0, 1636.0, 1641.0, 1646.0, 1651.0, 1656.0, 1661.0, 1665.0, 1670.0, 1675.0, 1680.0, 1685.0, 1690.0, 1695.0, 1700.0, 1704.0, 1709.0, 1714.0, 1719.0, 1724.0, 1729.0, 1734.0, 1738.0, 1743.0, 1748.0, 1753.0, 1758.0, 1763.0, 1768.0, 1772.0, 1777.0, 1782.0, 1787.0, 1792.0, 1797.0, 1802.0, 1806.0, 1811.0, 1816.0, 1821.0, 1826.0, 1831.0, 1836.0, 1840.0, 1845.0, 1850.0, 1855.0, 1860.0, 1865.0, 1869.0, 1874.0, 1879.0, 1884.0, 1889.0, 1894.0, 1898.0, 1903.0, 1908.0, 1913.0, 1918.0, 1923.0, 1927.0, 1932.0, 1937.0, 1942.0, 1947.0, 1952.0, 1956.0, 1961.0, 1966.0, 1971.0, 1976.0, 1981.0, 1985.0, 1990.0, 1995.0, 2000.0, 2005.0, 2009.0, 2014.0, 2019.0, 2024.0, 2029.0, 2034.0, 2038.0, 2043.0, 2048.0] ("Complete SkewTri")] -> w1
    frame "40MHz/32KHz", Default {
      # "40M"
      n2 = xnode "Open FPGA VI Reference"() -> ("FPGA VI Reference Out"=w68:refnum<k20>, "error out"=w67:errorcluster)  [unwired: 2 in]
    }
    frame "30MHz/24Khz" {
      # "30M"
      n3 = xnode "Open FPGA VI Reference"() -> ("FPGA VI Reference Out"=w71:refnum<k20>, "error out"=w72:errorcluster)  [unwired: 2 in]
    }
  }
  n4 = xnode "Invoke Method"("FPGA VI Reference In"=w34, "error in"=w33) -> ("FPGA VI Reference Out"=w31:refnum<k20>, "error out"=w32:errorcluster)
  n5 = xnode "Read/Write Control"("FPGA VI Reference In"=w31, "error in"=w32, "n"="#Signals") -> ("FPGA VI Reference Out"=w30:refnum<k20>, "error out"=w29:errorcluster)
  n6 = Add(x="lower limit 1", y=w60) -> (x+y=w64:u32)
  n7 = Add(x="lower limit 2", y=w60) -> (x+y=w62:u32)
  n8 = xnode "Read/Write Control"("FPGA VI Reference In"=w30, "error in"=w29, "upper limit 1"=w64, "upper limit 2"=w62, "lower limit 1"="lower limit 1", "lower limit 2"="lower limit 2", "Latency points"="Initial Latency points") -> ("FPGA VI Reference Out"=w58:refnum<k20>, "error out"=w57:errorcluster)
  n9 = xnode "Invoke Method"("FPGA VI Reference In"=w58, "error in"=w57, "Requested Depth"=u32 1000000) -> ("FPGA VI Reference Out"=w45:refnum<k20>, "error out"=w46:errorcluster)  [unwired: 1 out]
  n10 = xnode "Invoke Method"("FPGA VI Reference In"=w45, "error in"=w46, "Requested Depth"=u32 1000000) -> ("FPGA VI Reference Out"=w52:refnum<k20>, "error out"=w53:errorcluster)  [unwired: 1 out]
  n11 = xnode "Invoke Method"("FPGA VI Reference In"=w52, "error in"=w53) -> ("FPGA VI Reference Out"=w43:refnum<k20>, "error out"=w44:errorcluster)
  n12 = xnode "Invoke Method"("FPGA VI Reference In"=w43, "error in"=w44) -> ("FPGA VI Reference Out"=w38:refnum<k20>, "error out"=w51:errorcluster)
  n13 = xnode "Invoke Method"("FPGA VI Reference In"=w38, "error in"=w51) -> ("FPGA VI Reference Out"=w39:refnum<k20>, "error out"=w42:errorcluster)  [unwired: 1 in]
  n14 = To Long Integer(number="#Signals") -> (32bit integer=w19:i32)
  n15 = Multiply(x="#Signals", y=u32 1024 ("elements in array (1)")) -> (x*y=w14:u32)
  n16 = call "N-Wave Memory write from DMA - Host.vi"("Triangular Multiply Factor"="Triangular Multiply Factor", "Enable triangular scaling"="Enable triangular scaling", "n"=w19, "error in"=w42, "Custom Triangular Signal (fal-ris)"=w1, "Triangolo dritto?"="Triangolo dritto?", "FPGA VI Reference In"=w38) -> ("FPGA VI Reference Out"=w40:refnum<k20>, "error out"=w41:errorcluster)  [unwired: 2 in, 1 out]
  n17 = RT FIFO Create(1:dbl[] [] ("double precision float"), 4:u32 1000 ("size (10)"), 6:w14) -> (8:w11:refnum<k33>, 11:w12:errorcluster)  [unwired: 5 in, 1 out]
  n18 = call "Window Memory write from DMA - Host.vi"("error in"=w41, "Enum"="Windowing", "FPGA VI Reference In"=w40) -> ("error out"=w59:errorcluster)  [unwired: 5 in, 3 out]
  n19 = Multiply(x="#Signals", y=u32 1024 ("elements in array (1)")) -> (x*y=w23:u32)
  n20 = RT FIFO Create(1:dbl[] [] ("double precision float"), 4:u32 1000 ("size (10)"), 6:w23) -> (8:w6:refnum<k33>, 11:w20:errorcluster)  [unwired: 5 in, 1 out]
  n21 = node-c288(i64 10 ("Period")) -> (w37:T2)  [unwired: 3 in]
  n22 = while {
    tunnel: w11 -> [w87]
    tunnel: "first bin" -> [w84]
    tunnel: "last bin" -> [w83]
    tunnel: "Windowing" -> [w82]
    tunnel: "#Signals" -> [w81]
    shift-right: [w78] -> _
    shift-left: u32 0 ("#Signals") -> [w79]
    shift-right: [w75] -> _
    shift-left: w4 -> [w76]
    shift-right: [w74] -> _
    shift-left: w4 -> [w77]
    tunnel: w2 -> [w73]
    stop <- w80 stop-if-true
    n23 = Wait (ms)(milliseconds to wait=u32 10 ("millisecond multiple")) -> ()  [unwired: 1 out]
    n24 = RT FIFO Read(0:w87) -> (9:w85:dbl[], 10:w86:bool)  [unwired: 3 in, 3 out]
    n25 = case shown="False" w86 {
      tunnel: w85 -> [w125 _]
      tunnel: w84 -> [w121 _]
      tunnel: w83 -> [w120 _]
      tunnel: w82 -> [w119 _]
      tunnel: w81 -> [w115 _]
      tunnel: w79 -> [w104 w181]
      tunnel: [w93 w181] -> w78
      tunnel: w77 -> [w103 w179]
      tunnel: w76 -> [w102 w180]
      tunnel: [w95 w180] -> w75
      tunnel: [w96 w179] -> w74
      tunnel: w73 -> [w89 _]
      frame False {
        # "Calcolo del fattore correttivo\n(meglio farlo mediato)"
        n26 = Array Size(array=w125) -> (size(s)=w123:i32)
        n27 = Divide(x=w123, y=2) -> (x/y=w124:dbl)
        n28 = Split 1D Array(array=w125, index=w124) -> (first subarray=w117:dbl[], second subarray=w118:dbl[])
        n29 = while {
          shift-right: [w175] -> _
          shift-left: w117 -> [w178]
          shift-right: [w176] -> _
          shift-left: w118 -> [w177]
          tunnel: w121 -> [w172]
          tunnel: w120 -> [w171]
          tunnel: w119 -> [w162]
          tunnel: w89 -> [w159]
          tunnel: 512.0 ("FFT size") -> [w158]
          tunnel: [w157] -> w114 mode=indexing
          tunnel: [w156] -> w112 mode=indexing
          tunnel: w115 -> [w154]
          i -> [w151]
          stop <- w155 stop-if-true
          w153 = 256 ("x")
          n30 = Increment(x=w151) -> (x+1=w152:i32)
          n31 = Split 1D Array(array=w178, index=w153) -> (first subarray=w174:dbl[], second subarray=w175:dbl[])
          n32 = Split 1D Array(array=w177, index=w153) -> (first subarray=w173:dbl[], second subarray=w176:dbl[])
          n33 = Equal?(x=w152, y=w154) -> (x = y?=w155:bool)
          n34 = call "Max Bin Detection.vi"("FFT Array"=w174, "Init Discard Bins"=w172, "Last Discard Bins"=w171) -> ("Max Bin"=w170:i32, "Prev Max Amp"=w168:dbl, "Max Amp"=w169:dbl, "Succ Max Amp"=w167:dbl)  [unwired: 11 in, 2 out]
          n35 = call "Max Bin Detection.vi"("FFT Array"=w173, "Init Discard Bins"=w172, "Last Discard Bins"=w171) -> ("Max Bin"=w166:i32, "Prev Max Amp"=w164:dbl, "Max Amp"=w165:dbl, "Succ Max Amp"=w163:dbl)  [unwired: 11 in, 2 out]
          n36 = call "IFFT Bin interpolation.vi"("Max Bin"=w170, "Max Amp"=w169, "Prev Max Amp"=w168, "Succ Max Amp"=w167, "Windowing"=w162) -> ("Interpolate Bin"=w161:dbl)
          n37 = call "IFFT Bin interpolation.vi"("Max Bin"=w166, "Max Amp"=w165, "Prev Max Amp"=w164, "Succ Max Amp"=w163, "Windowing"=w162) -> ("Interpolate Bin"=w160:dbl)
          n38 = call "Frequency from bin number RT.vi"("FFT size"=w158, "Bin number"=w161, "Sample Rate (S/s)"=w159) -> ("Detected Frequency (Hz)"=w157:dbl)  [unwired: 8 in]
          n39 = call "Frequency from bin number RT.vi"("FFT size"=w158, "Bin number"=w160, "Sample Rate (S/s)"=w159) -> ("Detected Frequency (Hz)"=w156:dbl)  [unwired: 8 in]
        }
        "Frequencies 1" <- w114
        "Frequencies 2" <- w112
        n40 = Index Array(array=w114, index="indice della triangolare a fattore 1") -> (element=w90:dbl)
        n41 = disable-structure shown="Enabled" {
          disable-tunnel: [w128 w129] -> w113
          disable-tunnel: w112 -> [w127 _]
          disable-tunnel: "indice della triangolare a fattore 1" -> [w126 _]
          disable-tunnel: w90 -> [_ w129]
          frame Disabled {
            n42 = Index Array(array=w127, index=w126) -> (element=w128:dbl)
          }
          frame Enabled {
          }
        }
        n43 = Divide(x=w114, y=w90) -> (x/y=w101:dbl[])
        "Freq correction factor 1" <- w101
        n44 = Divide(x=w112, y=w113) -> (x/y=w100:dbl[])
        "Freq correction factor 2" <- w100
        n45 = Less Or Equal?(x=w101, y=1.0) -> (x <= y?=w109:bool[])
        n46 = Less Or Equal?(x=w100, y=1.0) -> (x <= y?=w108:bool[])
        n47 = And Array Elements(Boolean array=w109) -> (logical AND=w106:bool)
        n48 = And Array Elements(Boolean array=w108) -> (logical AND=w105:bool)
        n49 = And(x=w106, y=w105) -> (x .and. y?=w91:bool)
        n50 = case shown="True" w91 {
          tunnel: w104 -> [w142 w150]
          tunnel: [w142 w149] -> w94
          tunnel: w103 -> [w141 w147]
          tunnel: w102 -> [w140 w145]
          tunnel: w101 -> [_ w148]
          tunnel: w100 -> [_ w146]
          tunnel: [w140 w144] -> w97
          tunnel: [w141 w143] -> w98
          frame False {
          }
          frame True {
            n51 = Add(x=w146, y=w145) -> (x+y=w144:dbl[])
            n52 = Add(x=w148, y=w147) -> (x+y=w143:dbl[])
            n53 = Increment(x=w150) -> (x+1=w149:u32)
          }
        }
        "current sig factor" <- w94
        n54 = Equal?(x="#measure for factor", y=w94) -> (x = y?=w99:bool)
        n55 = case shown="True" w99 {
          tunnel: w98 -> [w132 w139]
          tunnel: w97 -> [w131 w138]
          tunnel: [w132 w134] -> w96
          tunnel: [w131 w134] -> w95
          tunnel: w94 -> [w130 w133]
          tunnel: [w130 u32 0 ("#Signals")] -> w93
          frame False {
          }
          frame True {
            w134 = dbl[] [0.0, 0.0, 0.0, 0.0, 0.0] ("second subarray")
            n56 = Divide(x=w139, y=w133) -> (x/y=→"mean factor 1":dbl[])
            n57 = Divide(x=w138, y=w133) -> (x/y=→"mean factor 2":dbl[])
          }
        }
      }
      frame True {
      }
    }
    n58 = local read "stop"() -> (w80:bool)
  }
  n59 = timed-loop {
    tunnel: w39 -> [w210]
    tunnel: w59 -> [w211]
    tunnel: [w213] -> w50
    tunnel: [w214] -> w49
    tunnel: [w199] -> w47
    tunnel: "#Signals" -> [w196]
    timing: w37 -> [_]
    timing-out: [_] -> w36
    tunnel: w6 -> [w194]
    shift-right: [w190] -> w21
    shift-left: w20 -> [w192]
    shift-right: [w186] -> _
    shift-left: 0 -> [w189]
    tunnel: w11 -> [w185]
    tunnel: w12 -> [w182]
    stop <- "stop" stop-if-true
    n60 = node-c288() -> ()  [unwired: 1 in, 1 out]
    n61 = flat-sequence {
      tunnel: w210 -> [w225]
      tunnel: w211 -> [w226]
      tunnel: "Snapshot" -> [w223]
      tunnel: "Snapshot" -> [w228]
      tunnel: [w227] -> w209
      tunnel: [w228] -> w208
      tunnel: [w223] -> w207
      tunnel: [w227] -> w206
      tunnel: [w224] -> w205
      tunnel: [w224] -> w204
      tunnel: [w222] -> w197
      tunnel: w196 -> [w222]
      tunnel: [w221] -> w195
      tunnel: w194 -> [w221]
      tunnel: [w220] -> w193
      tunnel: w192 -> [w220]
      tunnel: w189 -> [w219]
      tunnel: [w219] -> w188
      tunnel: w185 -> [w218]
      tunnel: [w218] -> w184
      tunnel: [w217] -> w183
      tunnel: w182 -> [w217]
      tunnel: w209 -> [w252]
      tunnel: w208 -> [w246]
      tunnel: w207 -> [w249]
      tunnel: w206 -> [w248]
      tunnel: w205 -> [w247]
      tunnel: w204 -> [w253]
      tunnel: [w251] -> w203
      tunnel: [w250] -> w202
      tunnel: [w245] -> w201
      tunnel: [w244] -> w198
      tunnel: w197 -> [w243]
      tunnel: w195 -> [w242]
      tunnel: w193 -> [w241]
      tunnel: [w240] -> w191
      tunnel: w188 -> [w238]
      tunnel: [w238] -> w187
      tunnel: w184 -> [w237]
      tunnel: w183 -> [w236]
      tunnel: [w353] -> w213
      tunnel: [w354] -> w214
      tunnel: w203 -> [w354]
      tunnel: w202 -> [w353]
      tunnel: w201 -> [w350]
      tunnel: [w352] -> w199
      tunnel: w198 -> [w352]
      tunnel: w191 -> [w351]
      tunnel: [w351] -> w190
      tunnel: w187 -> [w349]
      tunnel: [w348] -> w186
      frame #0 {
        n62 = case shown="False" w223 {
          tunnel: [w229 w235] -> w227
          tunnel: w226 -> [w229 w234]
          tunnel: w225 -> [w230 w233]
          tunnel: [w230 w232] -> w224
          frame False {
          }
          frame True {
            n63 = xnode "Read/Write Control"("FPGA VI Reference In"=w233, "error in"=w234, "snapshot"=TRUE) -> ("FPGA VI Reference Out"=w232:refnum<k20>, "error out"=w235:errorcluster)
          }
        }
      }
      frame #1 {
        n64 = flat-sequence {
          tunnel: w253 -> [w265]
          tunnel: w252 -> [w264]
          tunnel: w246 -> [w261]
          tunnel: [w263] -> w256
          tunnel: [w262] -> w255
          tunnel: [w261] -> w254
          tunnel: w243 -> [w260]
          tunnel: w242 -> [w259]
          tunnel: w241 -> [w258]
          tunnel: [w257] -> w239
          tunnel: [w307] -> w250
          tunnel: w256 -> [w309]
          tunnel: w255 -> [w308]
          tunnel: w254 -> [w306]
          tunnel: [w306] -> w245
          tunnel: [w305] -> w244
          tunnel: [w304] -> w240
          tunnel: w239 -> [w304]
          frame #0 {
            n65 = case shown="True" w261 {
              tunnel: w265 -> [w270 w298]
              tunnel: w264 -> [w269 w297]
              tunnel: [w268 w296] -> w262
              tunnel: [w267 w295] -> w263
              tunnel: w260 -> [_ w294]
              tunnel: w259 -> [_ w285]
              tunnel: w258 -> [w266 w284]
              tunnel: [w266 w283] -> w257
              frame False {
                n66 = disable-structure shown="Enabled" {
                  disable-tunnel: w270 -> [w277 w280]
                  disable-tunnel: w269 -> [w275 w279]
                  disable-tunnel: [w274 w279] -> w268
                  disable-tunnel: [w271 w280] -> w267
                  frame Disabled {
                    n67 = xnode "Invoke Method"("FPGA VI Reference In"=w277, "error in"=w275, "Number of Elements"=u32 0) -> ("FPGA VI Reference Out"=w273:refnum<k20>, "error out"=w272:errorcluster, "Elements Remaining"=w276:u32)  [unwired: 1 in, 1 out]
                    n68 = xnode "Invoke Method"("FPGA VI Reference In"=w273, "error in"=w272, "Number of Elements"=w276) -> ("FPGA VI Reference Out"=w271:refnum<k20>, "error out"=w274:errorcluster)  [unwired: 1 in, 2 out]
                  }
                  frame Enabled {
                  }
                }
              }
              frame True {
                n69 = Multiply(x=w294, y=u32 1024 ("Number of Elements")) -> (x*y=w288:u32)
                n70 = xnode "Invoke Method"("FPGA VI Reference In"=w298, "error in"=w297, "Number of Elements"=w288, "Timeout (ms)"=-1) -> ("FPGA VI Reference Out"=w291:refnum<k20>, "error out"=w290:errorcluster, "Data"=w293:fxp<+/-,12,12>[])  [unwired: 1 out]
                n71 = To Double Precision Float(number=w293) -> (double precision float=w281:dbl[])
                "N-Signals" <- w281
                n72 = xnode "Invoke Method"("FPGA VI Reference In"=w291, "error in"=w290, "Number of Elements"=u32 0) -> ("FPGA VI Reference Out"=w295:refnum<k20>, "error out"=w296:errorcluster, "Elements Remaining"=→"Elements Remaining Signal":u32)  [unwired: 1 in, 1 out]
                n73 = case shown="True" "Linearization?" {
                  tunnel: w285 -> [_ w303]
                  tunnel: w284 -> [w299 w302]
                  tunnel: [w299 w301] -> w283
                  tunnel: w281 -> [_ w300]
                  frame False {
                  }
                  frame True {
                    n74 = RT FIFO Write(0:w303, 1:w300, 3:w302) -> (11:w301:errorcluster)  [unwired: 2 in, 3 out]
                  }
                }
              }
            }
          }
          frame #1 {
            n75 = case shown="False" w306 {
              tunnel: [w311 w314] -> w307
              tunnel: w309 -> [w310 w315]
              tunnel: w308 -> [w311 w313]
              tunnel: [w310 w312] -> w305
              frame False {
              }
              frame True {
                n76 = xnode "Read/Write Control"("FPGA VI Reference In"=w315, "error in"=w313, "snapshot"=FALSE) -> ("FPGA VI Reference Out"=w312:refnum<k20>, "error out"=w314:errorcluster)
              }
            }
          }
        }
        n77 = case shown="True" w249 {
          tunnel: w247 -> [w319 w346]
          tunnel: w248 -> [w318 w347]
          tunnel: [w317 w345] -> w251
          tunnel: w243 -> [_ w333]
          tunnel: w237 -> [_ w330]
          tunnel: w236 -> [_ w329]
          frame False {
            n78 = disable-structure shown="Enabled" {
              disable-tunnel: w319 -> [w325 _]
              disable-tunnel: w318 -> [w322 w327]
              disable-tunnel: [w321 w327] -> w317
              frame Disabled {
                n79 = xnode "Invoke Method"("FPGA VI Reference In"=w325, "error in"=w322, "Number of Elements"=u32 0) -> ("FPGA VI Reference Out"=w323:refnum<k20>, "error out"=w320:errorcluster, "Elements Remaining"=w324:u32)  [unwired: 1 in, 1 out]
                n80 = xnode "Invoke Method"("FPGA VI Reference In"=w323, "error in"=w320, "Number of Elements"=w324) -> ("error out"=w321:errorcluster)  [unwired: 1 in, 3 out]
              }
              frame Enabled {
              }
            }
          }
          frame True {
            n81 = Multiply(x=w333, y=u32 1024 ("Number of Elements")) -> (x*y=w337:u32)
            n82 = xnode "Invoke Method"("FPGA VI Reference In"=w346, "error in"=w347, "Number of Elements"=w337, "Timeout (ms)"=-1) -> ("FPGA VI Reference Out"=w341:refnum<k20>, "error out"=w342:errorcluster, "Data"=w344:fxp<+,44,44>[])  [unwired: 1 out]
            n83 = To Double Precision Float(number=w344) -> (double precision float=w343:dbl[])
            n84 = Square Root(x=w343) -> (sqrt(x)=w334:dbl[])
            n85 = xnode "Invoke Method"("FPGA VI Reference In"=w341, "error in"=w342, "Number of Elements"=u32 0) -> ("error out"=w345:errorcluster, "Elements Remaining"=→"Elements Remaining FFT":u32)  [unwired: 1 in, 2 out]
            n86 = call "CleanCompleteFFTArray.vi"("Complete FFT Array"=w334, "FFT Size"=512, "#Signals"=w333) -> ("Second Edge Array"=w331:dbl[], "First Edge Array"=w332:dbl[])  [unwired: 7 in]
            "First Edge N-FFT" <- w332
            "Second Edge N-FFT" <- w331
            n87 = Build Array (concatenate)(w332, w331) -> (w328:dbl[])
            n88 = RT FIFO Write(0:w330, 1:w328, 3:w329) -> ()  [unwired: 2 in, 4 out]
          }
        }
      }
      frame #2 {
        n89 = case shown="False" w350 {
          tunnel: w349 -> [w355 w359]
          tunnel: [w355 w360] -> w348
          frame False {
          }
          frame True {
            n90 = Decrement(x="tieni premuto per") -> (x-1=w356:i32)
            n91 = Greater Or Equal?(x=w359, y=w356) -> (x >= y?=w358:bool)
            n92 = case shown="True" w358 {
              tunnel: w359 -> [w361 _]
              tunnel: [w362 0] -> w360
              frame False {
                n93 = Increment(x=w361) -> (x+1=w362:i32)
              }
              frame True {
                n94 = local write "Snapshot"(FALSE ("Snapshot")) -> ()
              }
            }
          }
        }
      }
    }
    n95 = node-c288() -> ()  [unwired: 1 in, 1 out]
  }
  n96 = while {
    tunnel: "first bin" -> [_]
    tunnel: "last bin" -> [_]
    tunnel: "Windowing" -> [_]
    tunnel: w6 -> [w375]
    shift-right: [w369] -> _
    shift-left: w20 -> [w374]
    tunnel: [w366] -> _
    tunnel: w19 -> [w366]
    tunnel: w2 -> [w370]
    shift-right: [w367] -> _
    shift-left: 0 ("first bin") -> [w368]
    stop <- w365 stop-if-true
    n97 = Wait (ms)(milliseconds to wait=u32 10 ("millisecond multiple")) -> ()  [unwired: 1 out]
    n98 = RT FIFO Read(0:w375, 3:w374) -> (9:w371:dbl[], 10:w373:bool, 11:w369:errorcluster)  [unwired: 2 in, 2 out]
    n99 = case shown="False" w373 {
      tunnel: w371 -> [w394 _]
      tunnel: w366 -> [w393 _]
      tunnel: w370 -> [w392 _]
      tunnel: w368 -> [w385 w460]
      tunnel: [w379 w460] -> w367
      tunnel: w366 -> [w376 _]
      frame False {
        # "#signals"
        n100 = while {
          tunnel: w394 -> [w451]
          shift-right: [w431] -> w389
          shift-left: dbl[] [] ("SubtractedSignal") -> [w434]
          tunnel: w393 -> [w446]
          tunnel: w392 -> [w439]
          shift-right: [w430] -> w388
          shift-left: dbl[] [] ("SubtractedSignal") -> [w433]
          i -> [w438]
          stop <- w442 stop-if-true
          w449 = 512 ("y")
          # "odd/even position"
          # "2n-1"
          n101 = Multiply(x=2, y=w446) -> (x*y=w444:i32)
          n102 = Decrement(x=w444) -> (x-1=w443:i32)
          n103 = Multiply(x=w438, y=w449) -> (x*y=w450:i32)
          n104 = Equal?(x=w438, y=w443) -> (x = y?=w442:bool)
          n105 = Array Subset(array=w451, index=w450, length=w449) -> (w448:dbl[])
          n106 = call "Poly Fitting.vi"("Poly Grade"=5.0, "Signal"=w448) -> ("SubtractedSignal"=w440:dbl[])  [unwired: 8 in, 1 out]
          n107 = Quotient & Remainder(x=w438, y=2) -> (x-y*floor(x/y)=w436:i32)  [unwired: 1 out]
          n108 = call "Sliding FFT.vi"("Sample Freq"=w439, "FFT Win Size"=128, "SubSmoothSignal"=w440) -> ("Freq samples"=w432:dbl[])  [unwired: 7 in, 1 out]
          n109 = Equal To 0?(x=w436) -> (x = 0?=w435:bool)
          n110 = case shown="True" w435 {
            tunnel: w434 -> [w453 w458]
            tunnel: w433 -> [w455 w456]
            tunnel: w432 -> [w454 w459]
            tunnel: [w453 w457] -> w431
            tunnel: [w452 w456] -> w430
            frame False {
              # "rising"
              n111 = Build Array (concatenate)(w455, w454) -> (w452:dbl[])
            }
            frame True {
              # "falling"
              n112 = Build Array (concatenate)(w458, w459) -> (w457:dbl[])
            }
          }
        }
        n113 = Increment(x=w385) -> (x+1=w381:i32)
        "Current Signal" <- w381
        n114 = Equal?(x=1, y=w381) -> (x = y?=w383:bool)
        n115 = feedback #1() -> (w386:T5)  [unwired: 1 in]
        n116 = feedback #2() -> (w387:T5)  [unwired: 1 in]
        n117 = case shown="False" w383 {
          tunnel: w388 -> [w424 w427]
          tunnel: w389 -> [w425 w429]
          tunnel: [w423 w426] -> w378
          tunnel: [w422 w428] -> w377
          tunnel: w387 -> [w421 _]
          tunnel: w386 -> [w420 _]
          frame False {
            n118 = Build Array (concatenate)(w421, w425) -> (w422:T5)
            n119 = Build Array (concatenate)(w420, w424) -> (w423:T5)
          }
          frame True {
            n120 = Build Array(w429) -> (w428:T5)
            n121 = Build Array(w427) -> (w426:T5)
          }
        }
        n122 = feedback-in #1(w378) -> ()
        n123 = feedback-in #2(w377) -> ()
        n124 = Equal?(x="# Measurements for Linearization", y=w381) -> (x = y?=w380:bool)
        n125 = case shown="True" w380 {
          tunnel: w381 -> [w395 _]
          tunnel: [w395 0] -> w379
          tunnel: w378 -> [_ w402]
          tunnel: w377 -> [_ w403]
          tunnel: w376 -> [_ w401]
          frame False {
          }
          frame True {
            # "FFTsize-FFTwinsize=512-128=384"
            n126 = Decrement(x=w401) -> (x-1=w400:i32)
            n127 = while {
              tunnel: w403 -> [w419]
              tunnel: w402 -> [w418]
              tunnel: w400 -> [w412]
              tunnel: [w408] -> w396 mode=indexing
              tunnel: [w407] -> w397 mode=indexing
              tunnel: [w406] -> w398 mode=indexing
              tunnel: [w405] -> w399 mode=indexing
              i -> [w413]
              stop <- w411 stop-if-true
              n128 = Multiply(x=384 ("# Measurements for Linearization 2"), y=w413) -> (x*y=w416:i32)
              n129 = Equal?(x=w413, y=w412) -> (x = y?=w411:bool)
              n130 = Add(x=w416, y=383) -> (x+y=w414:i32)
              n131 = Array Subset(array=w419, index (col)=w416, length (col)=w414) -> (w410:T5)  [unwired: 2 in]
              n132 = Array Subset(array=w418, index (col)=w416, length (col)=w414) -> (w409:T5)  [unwired: 2 in]
              n133 = call "Mean Freq Curves.vi"("Set of Freq samples"=w409) -> ("StdDev%"=w408:dbl, "Mean Freq Curve"=w406:dbl[])  [unwired: 9 in]
              n134 = call "Mean Freq Curves.vi"("Set of Freq samples"=w410) -> ("StdDev%"=w407:dbl, "Mean Freq Curve"=w405:dbl[])  [unwired: 9 in]
            }
            "First Mean Freq Curves" <- w399
            "Second Mean Freq Curves" <- w398
            "First Std Deviations %" <- w397
            "Second Std Deviations %" <- w396
          }
        }
      }
      frame True {
      }
    }
    n135 = local read "stop"() -> (w365:bool)
  }
  n136 = node-c288(w36) -> ()  [unwired: 1 out]
  n137 = Merge Errors(w49, w50, w21) -> (w54:errorcluster)
  n138 = flat-sequence {
    tunnel: w54 -> [w468]
    tunnel: w47 -> [w463]
    tunnel: w6 -> [w461]
    frame #0 {
      n139 = xnode "Invoke Method"("FPGA VI Reference In"=w463, "error in"=w468) -> ("FPGA VI Reference Out"=w465:refnum<k20>, "error out"=w464:errorcluster)
      n140 = RT FIFO Delete(0:w461) -> ()  [unwired: 2 in, 1 out]
      n141 = property on="stop" class="Bool (strict)"("Value"=FALSE ("stop")) -> ()  [unwired: 2 in, 2 out]
      n142 = xnode "Invoke Method"("FPGA VI Reference In"=w465, "error in"=w464) -> ("FPGA VI Reference Out"=w466:refnum<k20>, "error out"=w467:errorcluster)
      n143 = xnode "Close FPGA VI Reference"("FPGA VI Reference In"=w466, "error in"=w467) -> ()  [unwired: 1 out]
    }
  }
